vi "TestCopyARGBImageWithMask.vi"(8 "error in (no error)":errorcluster, 11 "Test Case In":refnum<class "Image.lvclass">) -> (0 "error out":errorcluster, 3 "Test Case Out":refnum<class "Image.lvclass">)   [LabVIEW 2020, in "g_ar_toolkit.test.lvlib" / "Image.lvclass"]
uses:
  Image.lvclass
  C:/Program Files (x86)/National Instruments/LabVIEW 2020/vi.lib/Astemes/LUnit/Test Case.lvclass
  g_ar_toolkit/Image Size Cluster.ctl
  <vilib>/Astemes/LUnit/Test Case.lvclass/Test Case.ctl
  g_ar_toolkit/Create_Empty_Image_ARGB.vi
  g_ar_toolkit/Copy_Image_ARGB_Mask_ARGB.vi
  4993e8ee-a06a-463a-9684-69129f64d5ce.vi
  <vilib>/Astemes/LUnit/Append Pass Result.vi
  <vilib>/Astemes/LUnit/Append Fail Result.vi
  <vilib>/Astemes/LUnit/Describe Comparison.vi
  <vilib>/Astemes/LUnit/Compare Variants.vi
  <vilib>/Astemes/LUnit/Variant to string.vi
  <vilib>/Utility/error.llb/Error Cluster From Error Code.vi
  <vilib>/picture/picture.llb/Draw Rectangle.vi
  <vilib>/picture/pictutil.llb/Picture to Pixmap.vi
  <vilib>/Utility/Data Type/Get Type Information.vi
  <vilib>/Utility/LVClass/Get LV Class Name.vi
  Image.lvclass/Image.ctl
  g_ar_toolkit.lvlib
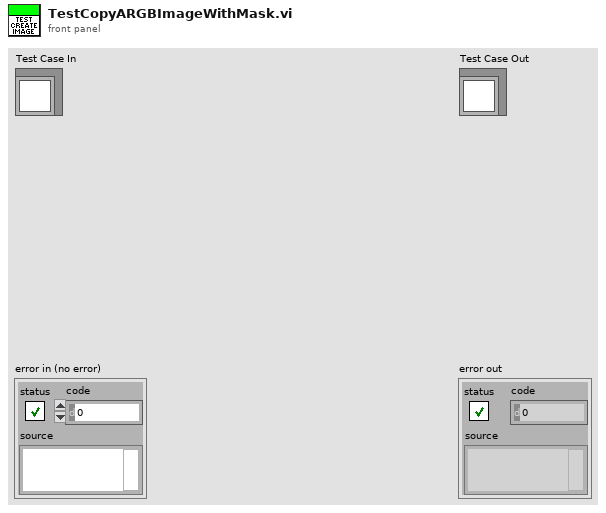
[diagram p1: front panel]
types:
  T1 = typedef "g_ar_toolkit.lvlib/Image Size Cluster.ctl" = cluster{"Width":u16, "Height":u16}
  T2 = typedef "imagedata.ctl" = cluster{"image type":i32, "image depth":i32, "image":u8[], "mask":u8[], "colors":u32[], "Rectangle":cluster{"left":i16, "top":i16, "right":i16, "bottom":i16}}
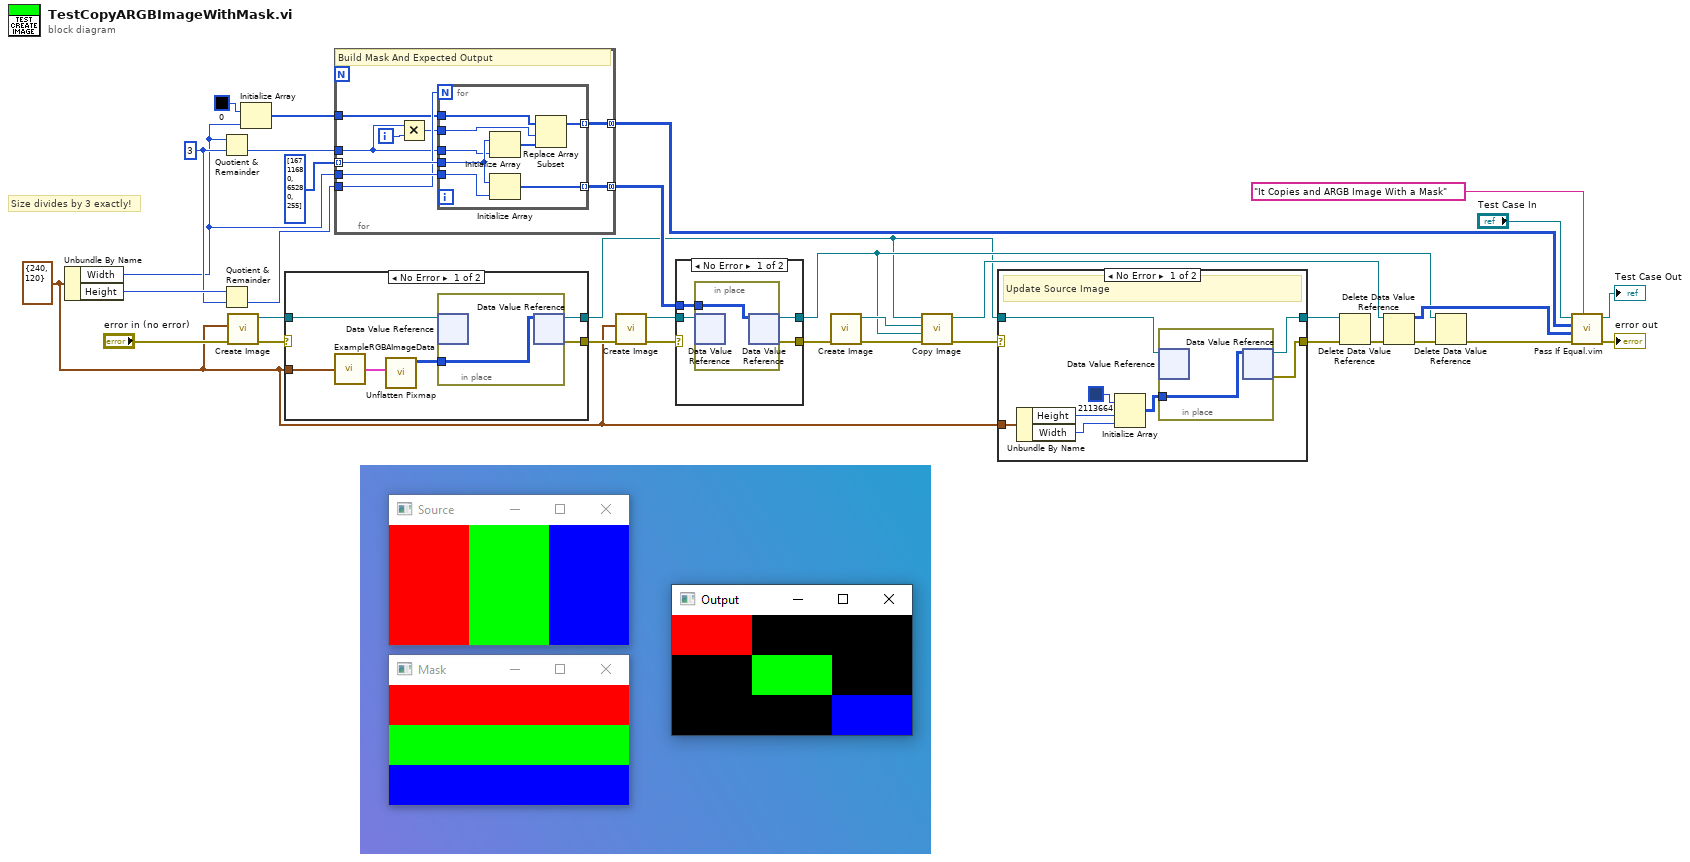
[diagram p0: block diagram]
diagram:
  w11 = u16 3 ("y")
  w1 = T1 {"Width"=240, "Height"=120} ("Preallocated Image Size (Default - 0,0)")
  # "Size divides by 3 exactly!"
  n1 = Unbundle By Name(w1) -> ("Width"=w5:u16, "Height"=w21:u16)
  n2 = Quotient & Remainder(x=w5, y=w11) -> (floor(x/y)=w10:u16)  [unwired: 1 out]
  n3 = Quotient & Remainder(x=w21, y=w11) -> (floor(x/y)=w20:u16)  [unwired: 1 out]
  n4 = call-poly "Create Image.vi"("error in (no error)"="error in (no error)", "Preallocated Image Size (Default - 0,0)"=w1) -> ("error out"=w28:errorcluster, "New ARGB Image"=w29:refnum<data-value>)  [unwired: 8 in]
  n5 = Initialize Array(u32 0, w5) -> (w3:u32[])
  n6 = case shown="No Error" w28 {
    selector: w28 -> [_ w42]
    tunnel: w29 -> [w40 w43]
    tunnel: [w39 w43] -> w7
    tunnel: [w38 w42] -> w6
    tunnel: w1 -> [w36 _]
    frame No Error {
      n7 = call "ExampleRGBAImageData.vi"("Image Size"=w36) -> ("RGB Image Data"=w35:T2)
      n8 = call <vilib>:"Unflatten Pixmap.vi"("image data"=w35) -> ("24-bit pixmap"=w37:u32[][])  [unwired: 4 in, 6 out]
      n9 = in-place {
        in-place-border: w37 -> [w41]
        n10 = in-place-dvr #1(w40) -> ()  [unwired: 2 out]
        n11 = in-place-dvr #1(w41) -> (w39:refnum<data-value>, w38:errorcluster)
      }
    }
    frame Error {
    }
  }
  n12 = for {
    tunnel: u32[] [16711680, 65280, 255] ("color(black)") -> [w52] mode=indexing
    tunnel: w5 -> [w51]
    tunnel: [w50] -> w19 mode=concatenating
    tunnel: w20 -> [w49]
    tunnel: w10 -> [w45]
    tunnel: w3 -> [w46]
    tunnel: [w44] -> w2 mode=concatenating
    i -> [w48]
    # "Build Mask And Expected Output"
    n13 = Multiply(x=w45, y=w48) -> (x*y=w47:i32)
    n14 = for {
      N: w49 -> [_]
      tunnel: w52 -> [w58]
      tunnel: w51 -> [w60]
      tunnel: [w59] -> w50 mode=indexing
      tunnel: w47 -> [w54]
      tunnel: w46 -> [w56]
      tunnel: w45 -> [w57]
      tunnel: [w53] -> w44 mode=indexing
      n15 = Initialize Array(w58, w57) -> (w55:u32[])
      n16 = Initialize Array(w58, w60) -> (w59:u32[])
      n17 = Replace Array Subset(array=w56, new element=w55, index=w54) -> (w53:u32[])
    }
  }
  n18 = call-poly "Create Image.vi"("error in (no error)"=w6, "Preallocated Image Size (Default - 0,0)"=w1) -> ("error out"=w17:errorcluster, "New ARGB Image"=w18:refnum<data-value>)  [unwired: 8 in]
  n19 = case shown="No Error" w17 {
    selector: w17 -> [_ w66]
    tunnel: w18 -> [w64 w67]
    tunnel: [w63 w67] -> w9
    tunnel: [w62 w66] -> w14
    tunnel: w19 -> [w61 _]
    frame No Error {
      n20 = in-place {
        in-place-border: w61 -> [w65]
        n21 = in-place-dvr #2(w64) -> ()  [unwired: 2 out]
        n22 = in-place-dvr #2(w65) -> (w63:refnum<data-value>, w62:errorcluster)
      }
    }
    frame Error {
    }
  }
  n23 = call-poly "Create Image.vi"("error in (no error)"=w14) -> ("error out"=w26:errorcluster, "New ARGB Image"=w27:refnum<data-value>)  [unwired: 9 in]
  n24 = call-poly "Copy Image.vi"("error in (no error)"=w26, "ARGB Image Mask"=w9, "ARGB Image Destination"=w27, "ARGB Image Source"=w7) -> ("error out"=w25:errorcluster, "ARGB Image Destination (duplicate)"=w13:refnum<data-value>)  [unwired: 6 in]
  n25 = case shown="No Error" w25 {
    selector: w25 -> [_ w77]
    tunnel: w7 -> [w75 w78]
    tunnel: [w74 w78] -> w24
    tunnel: [w73 w77] -> w8
    tunnel: w1 -> [w70 _]
    frame No Error {
      # "Update Source Image"
      n26 = Unbundle By Name(w70) -> ("Height"=w72:u16, "Width"=w71:u16)
      n27 = Initialize Array(u32 2113664, w72, w71) -> (w68:u32[][])
      n28 = in-place {
        in-place-border: w68 -> [w76]
        n29 = in-place-dvr #3(w75) -> ()  [unwired: 2 out]
        n30 = in-place-dvr #3(w76) -> (w74:refnum<data-value>, w73:errorcluster)
      }
    }
    frame Error {
    }
  }
  n31 = Delete Data Value Reference(data value reference=w24, error in=w8) -> (error out=w12:errorcluster)  [unwired: 1 out]
  n32 = Delete Data Value Reference(data value reference=w13, error in=w12) -> (data value=w23:u32[][], error out=w16:errorcluster)
  n33 = Delete Data Value Reference(data value reference=w9, error in=w16) -> (error out=w15:errorcluster)  [unwired: 1 out]
  n34 = call "Pass If Equal.vim"("Description"="It Copies and ARGB Image With a Mask", "error in (no error)"=w15, "Actual"=w23, "Expected"=w2, "LUnit Test Case In"="Test Case In") -> ("error out"=→"error out":errorcluster, "LUnit Test Case Out"=→"Test Case Out":refnum<class "Image.lvclass">)  [unwired: 5 in]
